vi "HWSyncLoop.vi"(5 "HAL":refnum<queue>, 6 "Index":u32, 7 "HWSync":refnum<queue>, 8 "error in":errorcluster, 9 "ACQ Data Queue":refnum<queue>, 10 "CTRL Data Notifier":refnum<notifier>, 11 "ACQ Data Notifier":refnum<notifier>) -> (0 "error out":errorcluster)   [LabVIEW 2014, in "HWSyncLoop.lvlib"]
uses:
  HWSyncLoop.lvlib
  APIs/Message Queue/Message Cluster.ctl
  APIs/Data Queue/Acquisition Data 1 Sample Cluster.ctl
  APIs/Data Queue/Control Data Cluster.ctl
  DriverMasterSync/build/DriverMasterSync.lvlibp/Modules/HAL/DriverMasterSync/DriverMasterSyncClass/DriverMasterSync.lvclass
  Typedefs/HWSync State.ctl
  <vilib>/Utility/error.llb/DialogType.ctl
  <vilib>/Utility/LVLibp/NI_PackedLibraryUtility.lvlib
  APIs/Message Queue/WINFAS 2 Message Queue.lvlib
  APIs/Data Queue/WINFAS 2 Data Queue.lvlib
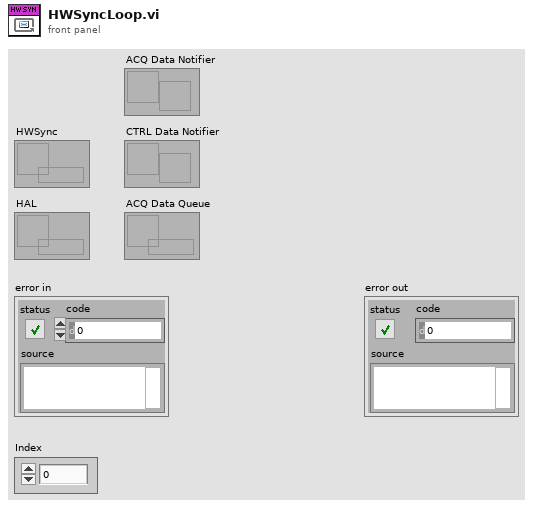
[diagram p1: front panel]
types:
  T1 = typedef "HWSyncLoop.lvlib/HWSync State.ctl" = enum16{"INIT", "Off", "Idle", "Auto-Refresh", "Sequence"}
  T2 = typedef "DialogType.ctl" = u16
  T3 = typedef "DriverMasterSync.lvlibp/HAL Config Data.ctl" = cluster{"HWSync Index":u32, "Driver Name":string, "Channel Mask":u64}
  T4 = typedef "DriverMasterSync.lvlibp/WINFAS 2 Data Queue.lvlib/Control Data Cluster.ctl" = cluster{"Encoder":sgl, "DI":bool[], "DO":bool[]}
  T5 = typedef "DriverMasterSync.lvlibp/WINFAS 2 Data Queue.lvlib/Acquisition Data 1 Sample Cluster.ctl" = cluster{"TDX":sgl[], "Encoder":sgl}
  T6 = typedef "DriverMasterSync.lvlibp/WINFAS 2 Data Queue.lvlib/Acquisition Data Cluster.ctl" = T5[]
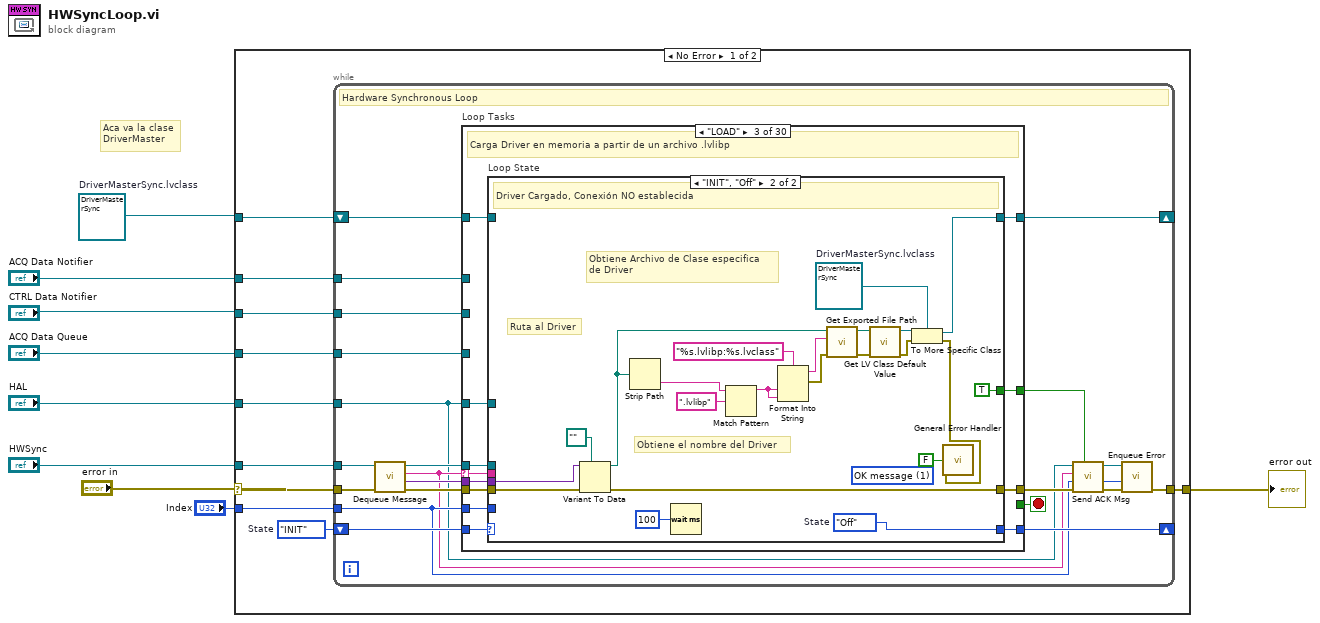
[diagram p0: block diagram]
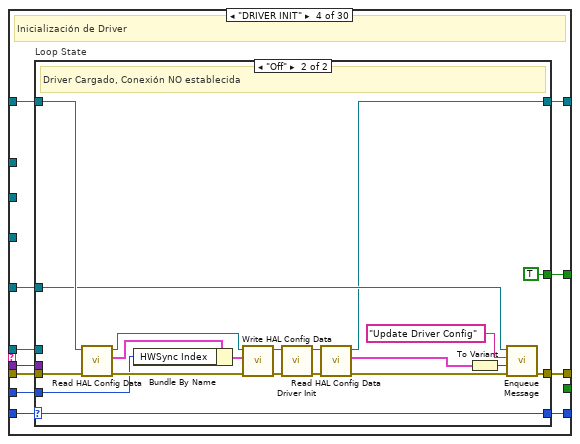
[diagram p5: hidden frame]
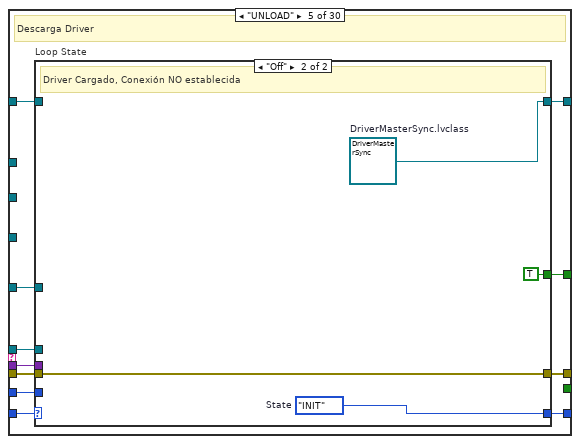
[diagram p7: hidden frame]
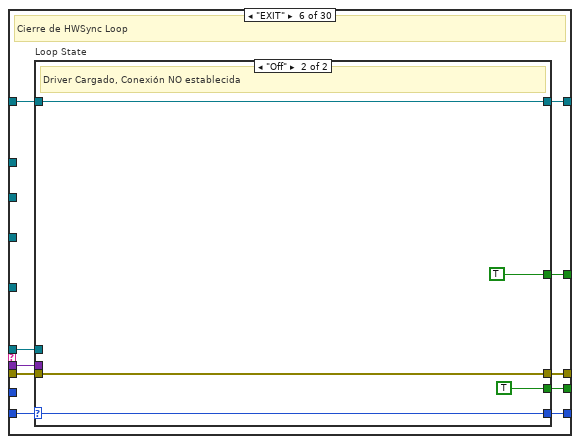
[diagram p9: hidden frame]
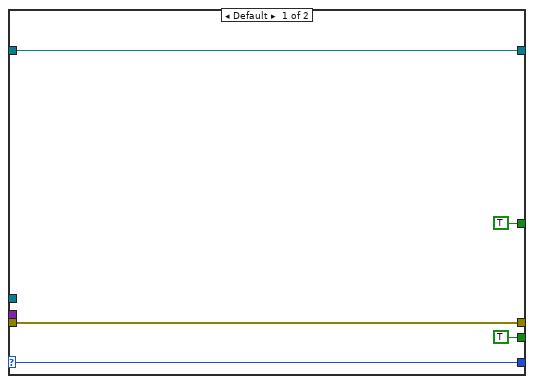
[diagram p10: hidden frame]
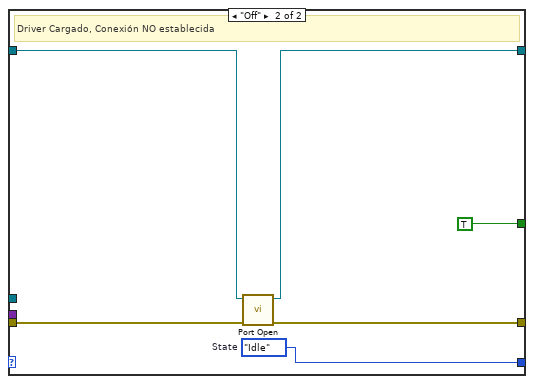
[diagram p13: hidden frame]
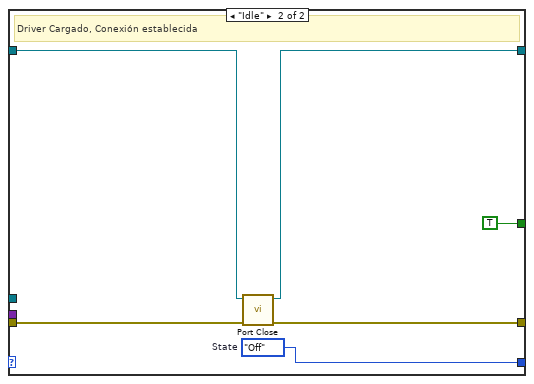
[diagram p15: hidden frame]
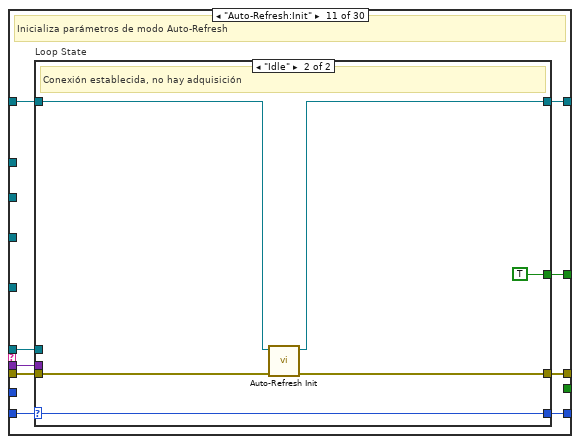
[diagram p17: hidden frame]
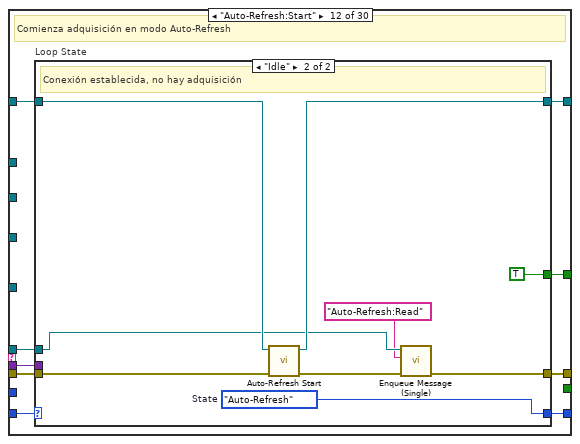
[diagram p19: hidden frame]
diagram:
  w5 = refnum<class "DriverMasterSync.lvclass"> refnum  # DriverMasterSync.lvclass
  # "Aca va la clase\nDriverMaster"
  n1 = case shown="No Error" "error in" {
    selector: "error in" -> [w19 w578]
    tunnel: [w15 w578] -> w8
    tunnel: "HWSync" -> [w18 _]
    tunnel: "HAL" -> [w16 _]
    tunnel: w5 -> [w14 _]
    tunnel: "Index" -> [w13 _]
    tunnel: "CTRL Data Notifier" -> [w12 _]
    tunnel: "ACQ Data Queue" -> [w11 _]
    tunnel: "ACQ Data Notifier" -> [w10 _]
    frame No Error {
      w17 = HWSync_State."INIT"  # State
      n2 = while {
        tunnel: w19 -> [w41]
        tunnel: w18 -> [w40]
        shift-right: [w35] -> _
        shift-left: w17 -> [w34]
        tunnel: w16 -> [w21]
        tunnel: [w30] -> w15
        shift-right: [w37] -> _
        shift-left: w14 -> [w29]
        tunnel: w13 -> [w23]
        tunnel: w12 -> [w33]
        tunnel: w11 -> [w32]
        tunnel: w10 -> [w31]
        stop <- w39 stop-if-true
        # "Hardware Synchronous Loop"
        n3 = call "Dequeue Message.vi"("error in (no error)"=w41, "Message Queue"=w40) -> ("error out"=w38:errorcluster, "Message Data"=w36:variant, "Message"=w22:string, "dup Message Queue"=w26:refnum<queue>)  [unwired: 6 in]
        n4 = case "Loop Tasks" shown="\"LOAD\"" w22 {
          selector: w22 -> [_ _ w49 _ _ _ _ _ _ _ _ _ _ _ _ _ _ _ _ _ _ _ _ _ _ _ _ _ _ _]
          tunnel: w26 -> [_ _ w55 w91 w125 w142 _ w164 w182 _ w203 w221 w243 w279 _ w302 w321 w345 w387 _ w408 w440 _ _ w473 w491 _ w513 w537 w558]
          tunnel: w21 -> [_ _ w50 w86 w120 _ _ _ _ _ _ _ _ _ _ _ _ _ _ _ _ _ _ _ _ _ _ w509 w533 w554]
          tunnel: [_ _ _ _ _ w138 _ _ _ _ _ _ _ _ _ _ _ _ _ _ _ _ _ _ _ _ _ _ _ _] -> w39
          tunnel: w38 -> [w44 w47 w58 w94 w128 w145 w159 w167 w185 w198 w206 w224 w246 w282 w297 w305 w324 w348 w390 w403 w411 w443 w462 w467 w476 w494 w507 w516 w540 w561]
          tunnel: [w44 w47 w56 w92 w126 w143 w159 w165 w183 w198 w204 w222 w244 w280 w297 w303 w322 w346 w388 w403 w409 w441 w462 w466 w474 w492 w507 w514 w538 w559] -> w28
          tunnel: w29 -> [w43 w46 w53 w89 w123 w140 w158 w162 w180 w197 w201 w219 w241 w277 w296 w300 w319 w343 w385 w402 w406 w438 w461 w465 w471 w489 w506 w511 w535 w556]
          tunnel: [w43 w46 w59 w95 w129 w146 w158 w168 w186 w197 w207 w225 w247 w283 w296 w306 w325 w349 w391 w402 w412 w444 w461 w464 w477 w495 w506 w517 w541 w562] -> w37
          tunnel: w36 -> [_ _ w57 w93 w127 w144 _ w166 w184 _ w205 w223 w245 w281 _ w304 w323 w347 w389 _ w410 w442 _ _ w475 w493 _ w515 w539 w560]
          tunnel: [w42 w45 w52 w88 w122 w139 w157 w161 w179 w196 w200 w218 w240 w276 w295 w299 w318 w342 w384 w401 w405 w437 w460 w468 w470 w488 w505 w510 w534 w555] -> w35
          tunnel: w34 -> [w42 w45 w54 w90 w124 w141 w157 w163 w181 w196 w202 w220 w242 w278 w295 w301 w320 w344 w386 w401 w407 w439 w460 w468 w472 w490 w505 w512 w536 w557]
          tunnel: w23 -> [_ _ w51 w87 w121 _ _ _ _ _ _ _ _ _ _ _ _ _ _ _ _ _ _ _ _ _ _ _ _ w552]
          tunnel: w33 -> [_ _ _ _ _ _ _ _ _ _ _ _ w239 w274 _ _ _ w340 _ _ _ _ _ _ _ _ _ _ _ _]
          tunnel: w32 -> [_ _ _ _ _ _ _ _ _ _ _ _ _ _ _ _ w316 w341 _ _ _ _ _ _ _ _ _ _ _ _]
          tunnel: w31 -> [_ _ _ _ _ _ _ _ _ _ _ _ w238 w275 _ _ _ w339 _ _ _ _ _ _ _ _ _ _ _ _]
          tunnel: [_ _ w48 w85 w119 w137 _ w160 w178 _ w199 w217 _ w273 _ w298 w317 _ w383 _ w404 w436 _ TRUE w469 w487 _ w508 w532 w553] -> w24
          frame "----LOOP----" {
          }
          frame Default {
          }
          frame "LOAD" {
            # "Carga Driver en memoria a partir de un archivo .lvlibp"
            n5 = case "Loop State" shown="\"INIT\", \"Off\"" w54 {
              selector: w54 -> [w60 _]
              tunnel: [w62 w78] -> w59
              tunnel: w58 -> [w61 w84]
              tunnel: w57 -> [_ w77]
              tunnel: [w61 w68] -> w56
              tunnel: w55 -> [_ _]
              tunnel: w53 -> [w62 _]
              tunnel: [w60 w70] -> w52
              tunnel: w51 -> [_ _]
              tunnel: w50 -> [_ _]
              tunnel: w49 -> [_ _]
              tunnel: [_ TRUE] -> w48
              frame Default {
              }
              frame "INIT", "Off" {
                (unwired) T2 1 items=["no dialog", "OK message", "continue or stop message", "OK message + warnings", "continue/stop + warnings"] ("type of dialog (OK msg:1)")
                w70 = HWSync_State."Off"  # State
                w79 = refnum<class "DriverMasterSync.lvclass"> refnum  # DriverMasterSync.lvclass
                # "Ruta al Driver"
                # "Obtiene el nombre del Driver"
                # "Obtiene Archivo de Clase especifica\nde Driver"
                # "Driver Cargado, Conexión NO establecida"
                n6 = Variant To Data(error in=w84, type=path "", Variant=w77) -> (data=w73:path, error out=w68:errorcluster)
                n7 = Strip Path(path=w73) -> (name=w74:string)  [unwired: 1 out]
                n8 = Wait (ms)(milliseconds to wait=u32 100) -> ()  [unwired: 1 out]
                n9 = Match Pattern(string=w74, regular expression=".lvlibp") -> (before substring=w72:string)  [unwired: 1 in, 3 out]
                n10 = Format Into String(format string="%s.lvlibp:%s.lvclass", w72, w72) -> (resulting string=w82:string, error out=w63:errorcluster)  [unwired: 2 in]
                n11 = call <vilib>:"Get Exported File Path.vi"("error in (no error)"=w63, "qualified name"=w82, "packed library path"=w73) -> ("error out"=w64:errorcluster, "path"=w83:path)  [unwired: 7 in]
                n12 = call <vilib>:"Get LV Class Default Value.vi"("error in (no error)"=w64, "class path"=w83) -> ("error out"=w65:errorcluster, "object"=w81:refnum<class>)  [unwired: 8 in]
                n13 = To More Specific Class(target class=w79, reference=w81, error in=w65) -> (specific class reference=w78:refnum<class "DriverMasterSync.lvclass">, error out=w66:errorcluster)
                n14 = call <vilib>:"General Error Handler.vi"("search ni.com link visible?(T)"=FALSE, "error in (no error)"=w66) -> ()  [unwired: 9 in, 5 out]
              }
            }
          }
          frame "DRIVER INIT" {
            # "Inicialización de Driver"
            n15 = case "Loop State" shown="\"Off\"" w90 {
              selector: w90 -> [w96 w118]
              tunnel: [w98 w103] -> w95
              tunnel: w94 -> [w97 w117]
              tunnel: w93 -> [_ _]
              tunnel: [w97 w108] -> w92
              tunnel: w91 -> [_ _]
              tunnel: w89 -> [w98 w116]
              tunnel: [w96 w118] -> w88
              tunnel: w87 -> [_ w109]
              tunnel: w86 -> [_ w107]
              tunnel: [_ TRUE] -> w85
              frame Default {
              }
              frame "Off" {
                # "Driver Cargado, Conexión NO establecida"
                n16 = call "Read HAL Config Data.vi"("error in (no error)"=w117, "DriverMasterSync in"=w116) -> ("error out"=w115:errorcluster, "HAL Config Data"=w111:T3, "DriverMasterSync out"=w113:refnum<class "DriverMasterSync.lvclass">)  [unwired: 7 in]
                n17 = Bundle By Name(cluster=w111, "HWSync Index"=w109) -> (w110:T3)
                n18 = call "Write HAL Config Data.vi"("error in (no error)"=w115, "HAL Config Data"=w110, "DriverMasterSync in"=w113) -> ("error out"=w114:errorcluster, "DriverMasterSync out"=w112:refnum<class "DriverMasterSync.lvclass">)  [unwired: 7 in]
                n19 = call-dynamic "Driver Init.vi"("error in (no error)"=w114, "DriverMasterSync in"=w112) -> ("error out"=w106:errorcluster, "DriverMasterSync out"=w104:refnum<class "DriverMasterSync.lvclass">)  [unwired: 8 in]
                n20 = call "Read HAL Config Data.vi"("error in (no error)"=w106, "DriverMasterSync in"=w104) -> ("error out"=w105:errorcluster, "HAL Config Data"=w100:T3, "DriverMasterSync out"=w103:refnum<class "DriverMasterSync.lvclass">)  [unwired: 7 in]
                n21 = To Variant(anything=w100) -> (Variant=w101:variant)
                n22 = call-poly "Enqueue Message.vi"("error in (no error)"=w105, "Message Data"=w101, "Message"="Update Driver Config", "Message Queue"=w107) -> ("error out"=w108:errorcluster)  [unwired: 6 in, 1 out]
              }
            }
          }
          frame "UNLOAD" {
            # "Descarga Driver"
            n23 = case "Loop State" shown="\"Off\"" w124 {
              selector: w124 -> [w130 _]
              tunnel: [w132 w133] -> w129
              tunnel: w128 -> [w131 w135]
              tunnel: w127 -> [_ _]
              tunnel: [w131 w135] -> w126
              tunnel: w125 -> [_ _]
              tunnel: w123 -> [w132 _]
              tunnel: [w130 w134] -> w122
              tunnel: w121 -> [_ _]
              tunnel: w120 -> [_ _]
              tunnel: [_ TRUE] -> w119
              frame Default {
              }
              frame "Off" {
                w133 = refnum<class "DriverMasterSync.lvclass"> refnum  # DriverMasterSync.lvclass
                w134 = HWSync_State."INIT"  # State
                # "Driver Cargado, Conexión NO establecida"
              }
            }
          }
          frame "EXIT" {
            # "Cierre de HWSync Loop"
            n24 = case "Loop State" shown="\"Off\"" w141 {
              selector: w141 -> [w149 w153]
              tunnel: [w151 w155] -> w146
              tunnel: w145 -> [w150 w154]
              tunnel: w144 -> [_ _]
              tunnel: [w150 w154] -> w143
              tunnel: w142 -> [_ _]
              tunnel: w140 -> [w151 w155]
              tunnel: [w149 w153] -> w139
              tunnel: [TRUE TRUE] -> w138
              tunnel: [TRUE TRUE] -> w137
              frame Default {
              }
              frame "Off" {
                # "Driver Cargado, Conexión NO establecida"
              }
            }
          }
          frame "----PORT----" {
          }
          frame "Port:Open" {
            # "Establece conexión con el Dispositivo"
            n25 = case "Loop State" shown="Default" w163 {
              selector: w163 -> [w169 _]
              tunnel: [w171 w176] -> w168
              tunnel: w167 -> [w170 w173]
              tunnel: w166 -> [_ _]
              tunnel: [w170 w175] -> w165
              tunnel: w164 -> [_ _]
              tunnel: w162 -> [w171 w177]
              tunnel: [w169 w174] -> w161
              tunnel: [_ TRUE] -> w160
              frame Default {
              }
              frame "Off" {
                w174 = HWSync_State."Idle"  # State
                # "Driver Cargado, Conexión NO establecida"
                n26 = call-dynamic "Port Open.vi"("error in (no error)"=w173, "DriverMasterSync in"=w177) -> ("error out"=w175:errorcluster, "DriverMasterSync out"=w176:refnum<class "DriverMasterSync.lvclass">)  [unwired: 8 in]
              }
            }
          }
          frame "Port:Close" {
            # "Finaliza conexión con el Dispositivo"
            n27 = case "Loop State" shown="Default" w181 {
              selector: w181 -> [w187 _]
              tunnel: [w189 w194] -> w186
              tunnel: w185 -> [w188 w191]
              tunnel: w184 -> [_ _]
              tunnel: [w188 w193] -> w183
              tunnel: w182 -> [_ _]
              tunnel: w180 -> [w189 w195]
              tunnel: [w187 w192] -> w179
              tunnel: [_ TRUE] -> w178
              frame Default {
              }
              frame "Idle" {
                w192 = HWSync_State."Off"  # State
                # "Driver Cargado, Conexión establecida"
                n28 = call-dynamic "Port Close.vi"("error in (no error)"=w191, "DriverMasterSync in"=w195) -> ("error out"=w193:errorcluster, "DriverMasterSync out"=w194:refnum<class "DriverMasterSync.lvclass">)  [unwired: 8 in]
              }
            }
          }
          frame "----AUTO-REFRESH----" {
          }
          frame "Auto-Refresh:Init" {
            # "Inicializa parámetros de modo Auto-Refresh"
            n29 = case "Loop State" shown="\"Idle\"" w202 {
              selector: w202 -> [w208 w216]
              tunnel: [w210 w214] -> w207
              tunnel: w206 -> [w209 w212]
              tunnel: w205 -> [_ _]
              tunnel: [w209 w213] -> w204
              tunnel: w203 -> [_ _]
              tunnel: w201 -> [w210 w215]
              tunnel: [w208 w216] -> w200
              tunnel: [_ TRUE] -> w199
              frame Default {
              }
              frame "Idle" {
                # "Conexión establecida, no hay adquisición"
                n30 = call-dynamic "Auto-Refresh Init.vi"("error in (no error)"=w212, "DriverMasterSync in"=w215) -> ("error out"=w213:errorcluster, "DriverMasterSync out"=w214:refnum<class "DriverMasterSync.lvclass">)  [unwired: 8 in]
              }
            }
          }
          frame "Auto-Refresh:Start" {
            # "Comienza adquisición en modo Auto-Refresh"
            n31 = case "Loop State" shown="\"Idle\"" w220 {
              selector: w220 -> [w226 _]
              tunnel: [w228 w235] -> w225
              tunnel: w224 -> [w227 w237]
              tunnel: w223 -> [_ _]
              tunnel: [w227 w233] -> w222
              tunnel: w221 -> [_ w232]
              tunnel: w219 -> [w228 w236]
              tunnel: [w226 w231] -> w218
              tunnel: [_ TRUE] -> w217
              frame Default {
              }
              frame "Idle" {
                w231 = HWSync_State."Auto-Refresh"  # State
                # "Conexión establecida, no hay adquisición"
                n32 = call-dynamic "Auto-Refresh Start.vi"("error in (no error)"=w237, "DriverMasterSync in"=w236) -> ("error out"=w234:errorcluster, "DriverMasterSync out"=w235:refnum<class "DriverMasterSync.lvclass">)  [unwired: 8 in]
                n33 = call "Enqueue Message (Single).vi"("error in (no error)"=w234, "Message"="Auto-Refresh:Read", "Message Queue"=w232) -> ("error out"=w233:errorcluster)  [unwired: 7 in, 1 out]
              }
            }
          }
          frame "Auto-Refresh:Read" {
            # "Realiza una lectura en modo Auto-Refresh"
            n34 = case "Loop State" shown="\"Auto-Refresh\"" w242 {
              selector: w242 -> [w248 w266]
              tunnel: [w250 w253] -> w247
              tunnel: w246 -> [w249 w265]
              tunnel: w245 -> [_ _]
              tunnel: [w249 w263] -> w244
              tunnel: w243 -> [_ w262]
              tunnel: w241 -> [w250 w264]
              tunnel: [w248 w266] -> w240
              tunnel: w239 -> [_ w260]
              tunnel: w238 -> [_ w258]
              frame Default {
              }
              frame "Auto-Refresh" {
                # "Adquiriendo en modo Auto-Refresh"
                n35 = for {
                  N: 1000 -> [_]
                  tunnel: [w269] -> w251
                  tunnel: [w268] -> w257
                  tunnel: w264 -> [w271]
                  tunnel: [w270] -> w253
                  tunnel: w265 -> [w272]
                  tunnel: [w267] -> w252
                  stop <- w267 continue-if-true
                  n36 = call-dynamic "Auto-Refresh Read.vi"("error in (no error)"=w272, "DriverMasterSync in"=w271) -> ("error out"=w267:errorcluster, "Control Data"=w268:T4, "1 Sample"=w269:T5, "DriverMasterSync out"=w270:refnum<class "DriverMasterSync.lvclass">)  [unwired: 6 in]
                }
                n37 = call "Send ACQ Notification.vi"("error in (no error)"=w252, "1 Sample"=w251, "ACQ Data Notifier in"=w258) -> ("error out"=w255:errorcluster)  [unwired: 7 in, 1 out]
                n38 = call "Send CTRL Notification.vi"("error in (no error)"=w252, "Control Data"=w257, "CTRL Data Notifier in"=w260) -> ("error out"=w256:errorcluster)  [unwired: 7 in, 1 out]
                n39 = Merge Errors(w255, w256) -> (w259:errorcluster)
                n40 = call "Enqueue Message (Single).vi"("error in (no error)"=w259, "Message"="Auto-Refresh:Read", "Message Queue"=w262) -> ("error out"=w263:errorcluster)  [unwired: 7 in, 1 out]
              }
            }
          }
          frame "Auto-Refresh:Stop" {
            # "Detiene adquisición en modo Auto-Refresh"
            n41 = case "Loop State" shown="\"Auto-Refresh\"" w278 {
              selector: w278 -> [w284 _]
              tunnel: [w286 w292] -> w283
              tunnel: w282 -> [w285 w294]
              tunnel: w281 -> [_ _]
              tunnel: [w285 w290] -> w280
              tunnel: w279 -> [_ _]
              tunnel: w277 -> [w286 w293]
              tunnel: [w284 w291] -> w276
              tunnel: w275 -> [_ w289]
              tunnel: w274 -> [_ w288]
              tunnel: [_ TRUE] -> w273
              frame Default {
              }
              frame "Auto-Refresh" {
                w291 = HWSync_State."Idle"  # State
                # "Adquiriendo en modo Auto-Refresh"
                n42 = Cancel Notification(0:w289) -> ()  [unwired: 1 in, 3 out]
                n43 = Cancel Notification(0:w288) -> ()  [unwired: 1 in, 3 out]
                n44 = call-dynamic "Auto-Refresh Stop.vi"("error in (no error)"=w294, "DriverMasterSync in"=w293) -> ("error out"=w290:errorcluster, "DriverMasterSync out"=w292:refnum<class "DriverMasterSync.lvclass">)  [unwired: 8 in]
              }
            }
          }
          frame "----SEQUENCE----" {
          }
          frame "Sequence:Init" {
            # "Inicializa parámetros de modo Sequence"
            n45 = case "Loop State" shown="\"Idle\"" w301 {
              selector: w301 -> [w307 w315]
              tunnel: [w309 w313] -> w306
              tunnel: w305 -> [w308 w311]
              tunnel: w304 -> [_ _]
              tunnel: [w308 w312] -> w303
              tunnel: w302 -> [_ _]
              tunnel: w300 -> [w309 w314]
              tunnel: [w307 w315] -> w299
              tunnel: [_ TRUE] -> w298
              frame Default {
              }
              frame "Idle" {
                # "Conexión establecida, no hay adquisición"
                n46 = call-dynamic "Sequence Init.vi"("error in (no error)"=w311, "DriverMasterSync in"=w314) -> ("error out"=w312:errorcluster, "DriverMasterSync out"=w313:refnum<class "DriverMasterSync.lvclass">)  [unwired: 8 in]
              }
            }
          }
          frame "Sequence:Start" {
            # "Comienza adquisición en modo Sequence"
            n47 = case "Loop State" shown="\"Idle\"" w320 {
              selector: w320 -> [w326 _]
              tunnel: [w328 w336] -> w325
              tunnel: w324 -> [w327 w338]
              tunnel: w323 -> [_ _]
              tunnel: [w327 w334] -> w322
              tunnel: w321 -> [_ w333]
              tunnel: w319 -> [w328 w337]
              tunnel: [w326 w332] -> w318
              tunnel: [_ TRUE] -> w317
              tunnel: w316 -> [_ w329]
              frame Default {
              }
              frame "Idle" {
                w332 = HWSync_State."Sequence"  # State
                # "Conexión establecida, no hay adquisición"
                n48 = Flush Queue(queue=w329) -> ()  [unwired: 1 in, 3 out]
                n49 = call-dynamic "Sequence Start.vi"("error in (no error)"=w338, "DriverMasterSync in"=w337) -> ("error out"=w335:errorcluster, "DriverMasterSync out"=w336:refnum<class "DriverMasterSync.lvclass">)  [unwired: 8 in]
                n50 = call "Enqueue Message (Single).vi"("error in (no error)"=w335, "Message"="Sequence:Read", "Message Queue"=w333) -> ("error out"=w334:errorcluster)  [unwired: 7 in, 1 out]
              }
            }
          }
          frame "Sequence:Read" {
            # "Realiza una lectura en modo Sequence"
            n51 = case "Loop State" shown="Default" w344 {
              selector: w344 -> [w350 w372]
              tunnel: [w352 w360] -> w349
              tunnel: w348 -> [w351 w371]
              tunnel: w347 -> [_ _]
              tunnel: [w351 w354] -> w346
              tunnel: w345 -> [_ w369]
              tunnel: w343 -> [w352 w370]
              tunnel: [w350 w372] -> w342
              tunnel: w341 -> [_ w366]
              tunnel: w340 -> [_ w365]
              tunnel: w339 -> [_ w363]
              frame Default {
              }
              frame "Sequence" {
                # "Adquiriendo en modo Sequence"
                n52 = for {
                  N: 1000 -> [_]
                  tunnel: [w375] -> w364
                  tunnel: [w374] -> w359
                  tunnel: w371 -> [w378]
                  tunnel: [w373] -> w356
                  tunnel: w370 -> [w377]
                  tunnel: [w376] -> w361
                  stop <- w373 continue-if-true
                  n53 = call-dynamic "Sequence Read.vi"("error in (no error)"=w378, "DriverMasterSync in"=w377) -> ("error out"=w373:errorcluster, "Control Data"=w375:T4, "Acquisition Data"=w374:T6, "DriverMasterSync out"=w376:refnum<class "DriverMasterSync.lvclass">)  [unwired: 6 in]
                }
                n54 = call-dynamic "Diagnostic Sample.vi"("error in (no error)"=w356, "Acquisition Data in"=w359, "DriverMasterSync in"=w361) -> ("error out"=w353:errorcluster, "Acquisition Data out"=w358:T6, "DriverMasterSync out"=w360:refnum<class "DriverMasterSync.lvclass">)  [unwired: 6 in]
                n55 = Index Array(array=w358) -> (element=w357:T5)  [unwired: 1 in]
                n56 = for {
                  tunnel: w366 -> [w382]
                  shift-right: [w380] -> w367
                  shift-left: w356 -> [w381]
                  tunnel: w358 -> [w379] mode=indexing
                  n57 = call "Enqueue ACQ Element.vi"("error in (no error)"=w381, "1 Sample"=w379, "ACQ Data Queue in"=w382) -> ("error out"=w380:errorcluster)  [unwired: 7 in, 1 out]
                }
                n58 = call "Send ACQ Notification.vi"("error in (no error)"=w356, "1 Sample"=w357, "ACQ Data Notifier in"=w363) -> ()  [unwired: 7 in, 2 out]
                n59 = call "Send CTRL Notification.vi"("error in (no error)"=w356, "Control Data"=w364, "CTRL Data Notifier in"=w365) -> ()  [unwired: 7 in, 2 out]
                n60 = call "Enqueue Message (Single).vi"("error in (no error)"=w367, "Message"="Sequence:Read", "Message Queue"=w369) -> ("error out"=w355:errorcluster)  [unwired: 7 in, 1 out]
                n61 = Merge Errors(w355, w353) -> (w354:errorcluster)
              }
            }
          }
          frame "Sequence:Stop" {
            # "Detiene adquisición en modo Sequence"
            n62 = case "Loop State" shown="\"Sequence\"" w386 {
              selector: w386 -> [w392 _]
              tunnel: [w394 w398] -> w391
              tunnel: w390 -> [w393 w400]
              tunnel: w389 -> [_ _]
              tunnel: [w393 w396] -> w388
              tunnel: w387 -> [_ _]
              tunnel: w385 -> [w394 w399]
              tunnel: [w392 w397] -> w384
              tunnel: [_ TRUE] -> w383
              frame Default {
              }
              frame "Sequence" {
                w397 = HWSync_State."Idle"  # State
                # "Adquiriendo en modo Sequence"
                n63 = call-dynamic "Sequence Stop.vi"("error in (no error)"=w400, "DriverMasterSync in"=w399) -> ("error out"=w396:errorcluster, "DriverMasterSync out"=w398:refnum<class "DriverMasterSync.lvclass">)  [unwired: 8 in]
              }
            }
          }
          frame "----OUTPUT----" {
          }
          frame "Digital Out Write" {
            # "Escribe el puerto de salidas digitales"
            n64 = case "Loop State" shown="\"Sequence\"" w407 {
              selector: w407 -> [w413 w417 w427]
              tunnel: [w415 w424 w434] -> w412
              tunnel: w411 -> [w414 w423 w433]
              tunnel: w410 -> [_ w421 w431]
              tunnel: [w414 w418 w428] -> w409
              tunnel: w408 -> [_ _ _]
              tunnel: w406 -> [w415 w425 w435]
              tunnel: [w413 w417 w427] -> w405
              tunnel: [_ TRUE TRUE] -> w404
              frame Default {
              }
              frame "Auto-Refresh" {
                # "Adquiriendo en modo Auto-Refresh"
                n65 = Variant To Data(error in=w423, type=u64 0, Variant=w421) -> (data=w419:u64, error out=w422:errorcluster)
                n66 = call-dynamic "Digital Out Write.vi"("error in (no error)"=w422, "Port Mask"=w419, "DriverMasterSync in"=w425) -> ("error out"=w418:errorcluster, "DriverMasterSync out"=w424:refnum<class "DriverMasterSync.lvclass">)  [unwired: 7 in]
              }
              frame "Sequence" {
                # "Adquiriendo en modo Sequence"
                n67 = Variant To Data(error in=w433, type=u64 0, Variant=w431) -> (data=w429:u64, error out=w432:errorcluster)
                n68 = call-dynamic "Digital Out Write.vi"("error in (no error)"=w432, "Port Mask"=w429, "DriverMasterSync in"=w435) -> ("error out"=w428:errorcluster, "DriverMasterSync out"=w434:refnum<class "DriverMasterSync.lvclass">)  [unwired: 7 in]
              }
            }
          }
          frame "Encoder Zero" {
            # "Resetea a cero el valor del encoder"
            n69 = case "Loop State" shown="Default" w439 {
              selector: w439 -> [w445 w450 w456]
              tunnel: [w447 w452 w458] -> w444
              tunnel: w443 -> [w446 w449 w455]
              tunnel: w442 -> [_ _ _]
              tunnel: [w446 w451 w457] -> w441
              tunnel: w440 -> [_ _ _]
              tunnel: w438 -> [w447 w453 w459]
              tunnel: [w445 w450 w456] -> w437
              tunnel: [_ TRUE TRUE] -> w436
              frame Default {
              }
              frame "Auto-Refresh" {
                # "Adquiriendo en modo Auto-Refresh"
                n70 = call-dynamic "Encoder Zero.vi"("error in (no error)"=w449, "DriverMasterSync in"=w453) -> ("error out"=w451:errorcluster, "DriverMasterSync out"=w452:refnum<class "DriverMasterSync.lvclass">)  [unwired: 8 in]
              }
              frame "Sequence" {
                # "Adquiriendo en modo Sequence"
                n71 = call-dynamic "Encoder Zero.vi"("error in (no error)"=w455, "DriverMasterSync in"=w459) -> ("error out"=w457:errorcluster, "DriverMasterSync out"=w458:refnum<class "DriverMasterSync.lvclass">)  [unwired: 8 in]
              }
            }
          }
          frame "----DIAGNOSTIC----" {
          }
          frame "Diagnostic:PowerON" {
            # "Diagnostico de Encendido"
            n72 = call-dynamic "Diagnostic Power ON.vi"("error in (no error)"=w467, "DriverMasterSync in"=w465) -> ("error out"=w466:errorcluster, "DriverMasterSync out"=w464:refnum<class "DriverMasterSync.lvclass">)  [unwired: 8 in]
          }
          frame "Diagnostic:Cycle" {
            # "Diagnostico de Comienzo de Ciclo"
            n73 = case "Loop State" shown="\"Auto-Refresh\"" w472 {
              selector: w472 -> [w478 w483]
              tunnel: [w480 w484] -> w477
              tunnel: w476 -> [w479 w486]
              tunnel: w475 -> [_ _]
              tunnel: [w479 w482] -> w474
              tunnel: w473 -> [_ _]
              tunnel: w471 -> [w480 w485]
              tunnel: [w478 w483] -> w470
              tunnel: [_ TRUE] -> w469
              frame Default {
              }
              frame "Auto-Refresh" {
                # "Adquiriendo en modo Auto-Refresh"
                n74 = call-dynamic "Diagnostic Cycle.vi"("error in (no error)"=w486, "DriverMasterSync in"=w485) -> ("error out"=w482:errorcluster, "DriverMasterSync out"=w484:refnum<class "DriverMasterSync.lvclass">)  [unwired: 8 in]
              }
            }
          }
          frame "Diagnostic:Measurement" {
            # "Diagnostico de Medición"
            n75 = case "Loop State" shown="\"Sequence\"" w490 {
              selector: w490 -> [w496 w501]
              tunnel: [w498 w502] -> w495
              tunnel: w494 -> [w497 w504]
              tunnel: w493 -> [_ _]
              tunnel: [w497 w500] -> w492
              tunnel: w491 -> [_ _]
              tunnel: w489 -> [w498 w503]
              tunnel: [w496 w501] -> w488
              tunnel: [_ TRUE] -> w487
              frame Default {
              }
              frame "Sequence" {
                # "Adquiriendo en modo Sequence"
                n76 = call-dynamic "Diagnostic Measurement.vi"("error in (no error)"=w504, "DriverMasterSync in"=w503) -> ("error out"=w500:errorcluster, "DriverMasterSync out"=w502:refnum<class "DriverMasterSync.lvclass">)  [unwired: 8 in]
              }
            }
          }
          frame "----UTILITY----" {
          }
          frame "Config" {
            # "Abre Panel de Configuración de Driver"
            n77 = case "Loop State" shown="\"Off\"" w512 {
              selector: w512 -> [w518 w529]
              tunnel: [w520 w530] -> w517
              tunnel: w516 -> [w519 w528]
              tunnel: w515 -> [_ _]
              tunnel: [w519 w526] -> w514
              tunnel: w513 -> [_ _]
              tunnel: w511 -> [w520 w531]
              tunnel: [w518 w529] -> w510
              tunnel: w509 -> [_ w525]
              tunnel: [_ TRUE] -> w508
              frame Default {
              }
              frame "Off" {
                # "HAL Config Data"
                # "Driver Cargado, Conexión NO establecida"
                n78 = call-dynamic "Config.vi"("error in (no error)"=w528, "DriverMasterSync in"=w531) -> ("error out"=w527:errorcluster, "HAL Config Data"=w522:T3, "DriverMasterSync out"=w530:refnum<class "DriverMasterSync.lvclass">)  [unwired: 7 in]
                n79 = To Variant(anything=w522) -> (Variant=w523:variant)
                n80 = call-poly "Enqueue Message.vi"("error in (no error)"=w527, "Message Data"=w523, "Message"="Update Driver Config", "Message Queue"=w525) -> ("error out"=w526:errorcluster)  [unwired: 6 in, 1 out]
              }
            }
          }
          frame "Config:Set" {
            # "Setea Configuración desde afuera"
            n81 = case "Loop State" shown="\"Off\"" w536 {
              selector: w536 -> [w542 w549]
              tunnel: [w544 w550] -> w541
              tunnel: w540 -> [w543 w548]
              tunnel: w539 -> [_ w545]
              tunnel: [w543 w546] -> w538
              tunnel: w537 -> [_ _]
              tunnel: w535 -> [w544 w551]
              tunnel: [w542 w549] -> w534
              tunnel: w533 -> [_ _]
              tunnel: [_ TRUE] -> w532
              frame Default {
              }
              frame "Off" {
                # "Driver Cargado, Conexión NO establecida"
                n82 = call-dynamic "Set Config.vi"("error in (no error)"=w548, "Config Data"=w545, "DriverMasterSync in"=w551) -> ("error out"=w546:errorcluster, "DriverMasterSync out"=w550:refnum<class "DriverMasterSync.lvclass">)  [unwired: 7 in]
              }
            }
          }
          frame "Config:Get" {
            # "Envía Configuración hacia afuera"
            n83 = case "Loop State" shown="\"Off\"" w557 {
              selector: w557 -> [w563 w575]
              tunnel: [w565 w576] -> w562
              tunnel: w561 -> [w564 w574]
              tunnel: w560 -> [_ _]
              tunnel: [w564 w571] -> w559
              tunnel: w558 -> [_ _]
              tunnel: w556 -> [w565 w577]
              tunnel: [w563 w575] -> w555
              tunnel: w554 -> [_ w570]
              tunnel: [_ TRUE] -> w553
              tunnel: w552 -> [_ w568]
              frame Default {
              }
              frame "Off" {
                # "Driver Cargado, Conexión NO establecida"
                n84 = call-dynamic "Get Config.vi"("error in (no error)"=w574, "DriverMasterSync in"=w577) -> ("error out"=w572:errorcluster, "Config Data"=w566:variant, "DriverMasterSync out"=w576:refnum<class "DriverMasterSync.lvclass">)  [unwired: 7 in]
                n85 = Format Into String(format string="CONFIG:HWSync:%d" ("Message"), w568) -> (resulting string=w567:string)  [unwired: 2 in, 1 out]
                n86 = call-poly "Enqueue Message.vi"("error in (no error)"=w572, "Message Data"=w566, "Message"=w567, "Message Queue"=w570) -> ("error out"=w571:errorcluster)  [unwired: 6 in, 1 out]
              }
            }
          }
        }
        n87 = call "Send ACK Msg.vi"("Enable?"=w24, "error in (no error)"=w28, "Index"=w23, "Message"=w22, "HAL  in"=w21) -> ("error out"=w27:errorcluster, "dup Index"=w20:u32, "HAL  out"=w25:refnum<queue>)  [unwired: 4 in]
        n88 = call "Enqueue Error.vi"("Error In"=w27, "Index"=w20, "HWSync Message Queue"=w25) -> ("dup Error Out"=w30:errorcluster)  [unwired: 8 in]
      }
    }
    frame Error {
    }
  }
  "error out" <- w8
